vi "Dual time calibration data preprocessing.vi"(0 "t0_U_cal t0 (m/s)":dbl[](array[numeric]), 1 "t0_Vout_cal t0 (V)":dbl[](array[numeric]), 5 "t0_Ta_cal (°C)":dbl[](array[numeric]), 7 "t1_Vout_cal t0 (V)":dbl[](array[numeric]), 9 "t1_U_cal t0 (m/s)":dbl[](array[numeric]), 11 "t1_Ta_cal (°C)":dbl[](array[numeric]), 12 "Overheat ratio":dbl=1.7, 13 "Gain":dbl=10.0, 14 "Offset (V)":dbl=0.512) -> (4 "t0 Calibration data":T1, 6 "t1* Calibration data":T1)   [LabVIEW 2022 SP3]
uses:
  Ctls/Calibration data.ctl
panel:
  out "Calibration curves":cluster{dbl[], dbl[]}[](graph)
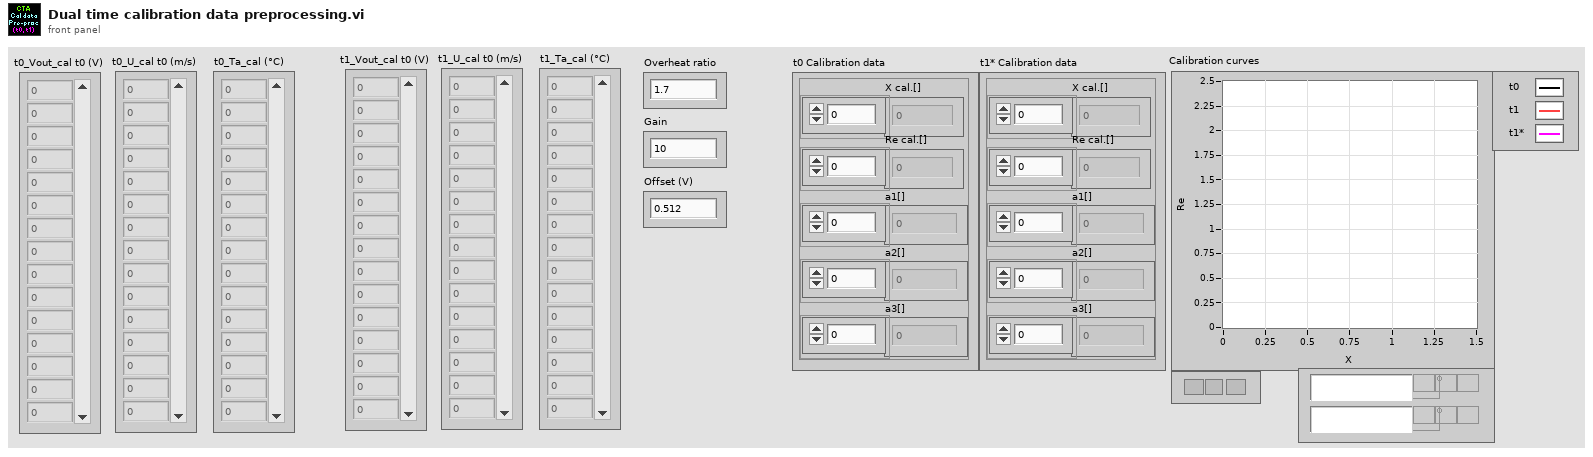
[diagram p1: front panel]
types:
  T1 = typedef "Calibration data.ctl" = cluster{"X cal.[]":dbl[], "Re cal.[]":dbl[], "a1[]":dbl[], "a2[]":dbl[], "a3[]":dbl[]}
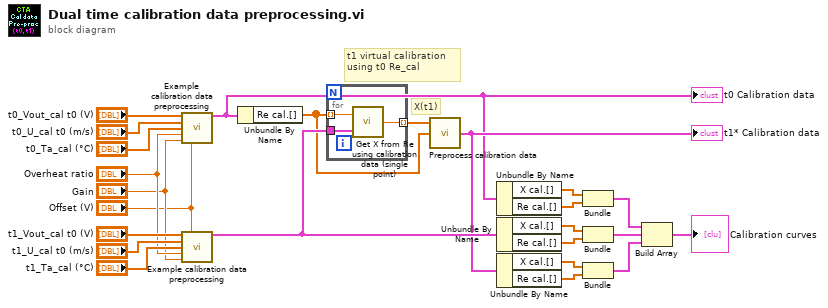
[diagram p0: block diagram]
diagram:
  # "t1 virtual calibration using t0 Re_cal"
  # "X(t1)"
  n1 = call "Example calibration data preprocessing.vi"("Vout_cal (V)"="t0_Vout_cal t0 (V)", "U_cal (m/s)"="t0_U_cal t0 (m/s)", "Ta_cal (°C)"="t0_Ta_cal (°C)", "Overheat ratio"="Overheat ratio", "Gain"="Gain", "Offset (V)"="Offset (V)") -> ("Calibration data"=w1:T1)  [unwired: 9 in]
  "t0 Calibration data" <- w1
  n2 = call "Example calibration data preprocessing.vi"("Vout_cal (V)"="t1_Vout_cal t0 (V)", "U_cal (m/s)"="t1_U_cal t0 (m/s)", "Ta_cal (°C)"="t1_Ta_cal (°C)", "Overheat ratio"="Overheat ratio", "Gain"="Gain", "Offset (V)"="Offset (V)") -> ("Calibration data"=w5:T1)  [unwired: 9 in]
  n3 = Unbundle By Name(w1) -> ("Re cal.[]"=w3:dbl[])
  n4 = for {
    tunnel: w3 -> [w27] mode=indexing
    tunnel: w5 -> [w26]
    tunnel: [w25] -> w4 mode=indexing
    n5 = call "Get X from Re using calibration data (single point).vi"("Calibration data"=w26, "Re"=w27) -> ("X"=w25:dbl)
  }
  n6 = call "Preprocess calibration data.vi"("Re cal.[]"=w3, "X cal.[]"=w4) -> ("Calibration data"=w2:T1)  [unwired: 1 in]
  "t1* Calibration data" <- w2
  n7 = Unbundle By Name(w1) -> ("X cal.[]"=w13:dbl[], "Re cal.[]"=w12:dbl[])
  n8 = Unbundle By Name(w5) -> ("X cal.[]"=w11:dbl[], "Re cal.[]"=w10:dbl[])
  n9 = Unbundle By Name(w2) -> ("X cal.[]"=w7:dbl[], "Re cal.[]"=w8:dbl[])
  n10 = Bundle("X cal.[]"=w13, "Re cal.[]"=w12) -> (w24:cluster{"X cal.[]":dbl[], "Re cal.[]":dbl[]})  [unwired: 1 in]
  n11 = Bundle("X cal.[]"=w11, "Re cal.[]"=w10) -> (w23:cluster{"X cal.[]":dbl[], "Re cal.[]":dbl[]})  [unwired: 1 in]
  n12 = Bundle("X cal.[]"=w7, "Re cal.[]"=w8) -> (w6:cluster{"X cal.[]":dbl[], "Re cal.[]":dbl[]})  [unwired: 1 in]
  n13 = Build Array(w24, w23, w6) -> (→"Calibration curves":cluster{"X cal.[]":dbl[], "Re cal.[]":dbl[]}[])
